vi "execute.vi"(8 "error in (no error)":errorcluster, 10 "Context in":refnum<class "Context.lvclass">, 11 "ApplyAOSCorrectionByBendingModesCommand in":refnum<class "ApplyAOSCorrectionByBendingModesCommand.lvclass">) -> (0 "error out":errorcluster, 2 "Context out":refnum<class "Context.lvclass">, 3 "ApplyAOSCorrectionByBendingModesCommand out":refnum<class "ApplyAOSCorrectionByBendingModesCommand.lvclass">)   [LabVIEW 2016, in "ApplyAOSCorrectionByBendingModesCommand.lvclass"]
uses:
  ApplyAOSCorrectionByBendingModesCommand.lvclass
  Context/Context.lvclass
  ApplyAOSCorrectionByBendingModesCommand.lvclass/ApplyAOSCorrectionByBendingModesCommand.ctl
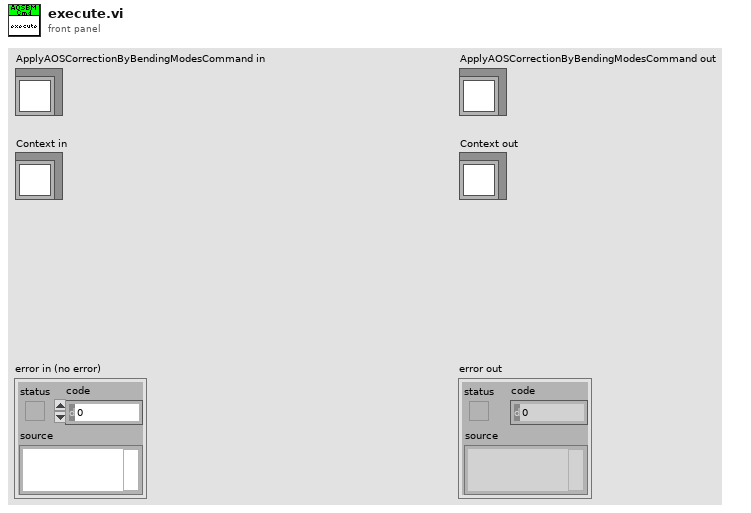
[diagram p1: front panel]
types:
  T1 = typedef "M1M3SupportTopics.lvlib/CommandApplyAOSCorrectionByBendingModes.ctl" = cluster{"CommandId":T2, "Coefficients":dbl[]}
  T2 = typedef "M1M3SupportTopics.lvlib/CommandId.ctl" = i32
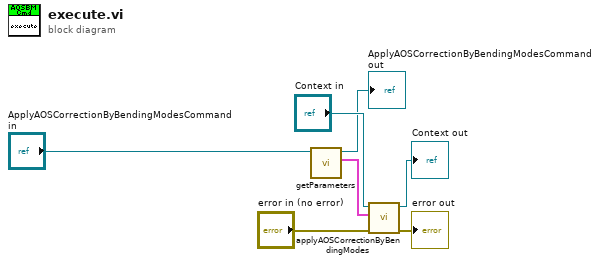
[diagram p0: block diagram]
diagram:
  n1 = call "getParameters.vi"("ApplyAOSCorrectionByBendingModesCommand in"="ApplyAOSCorrectionByBendingModesCommand in") -> ("Parameters"=w5:T1, "ApplyAOSCorrectionByBendingModesCommand out"=→"ApplyAOSCorrectionByBendingModesCommand out":refnum<class "ApplyAOSCorrectionByBendingModesCommand.lvclass">)  [unwired: 9 in]
  n2 = call-dynamic "applyAOSCorrectionByBendingModes.vi"("error in (no error)"="error in (no error)", "Parameters"=w5, "Context in"="Context in") -> ("error out"=→"error out":errorcluster, "Context out"=→"Context out":refnum<class "Context.lvclass">)  [unwired: 7 in]
